vi "RedoCurveFits.vi"() -> ()   [LabVIEW 2020]
uses:
  <vilib>/Utility/file.llb/Read Delimited Spreadsheet (DBL).vi
  <vilib>/Utility/file.llb/Write Delimited Spreadsheet (DBL).vi
panel:
  out "XY Graph 5":cluster{dbl[], dbl[]}[](graph)
  out "error out":errorcluster
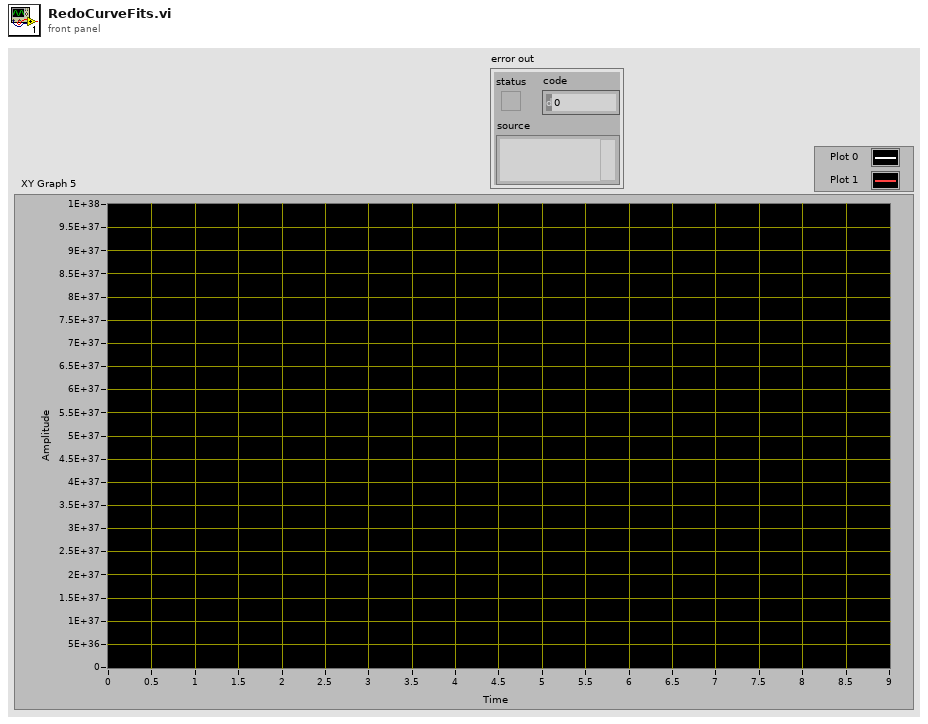
[diagram p1: front panel]
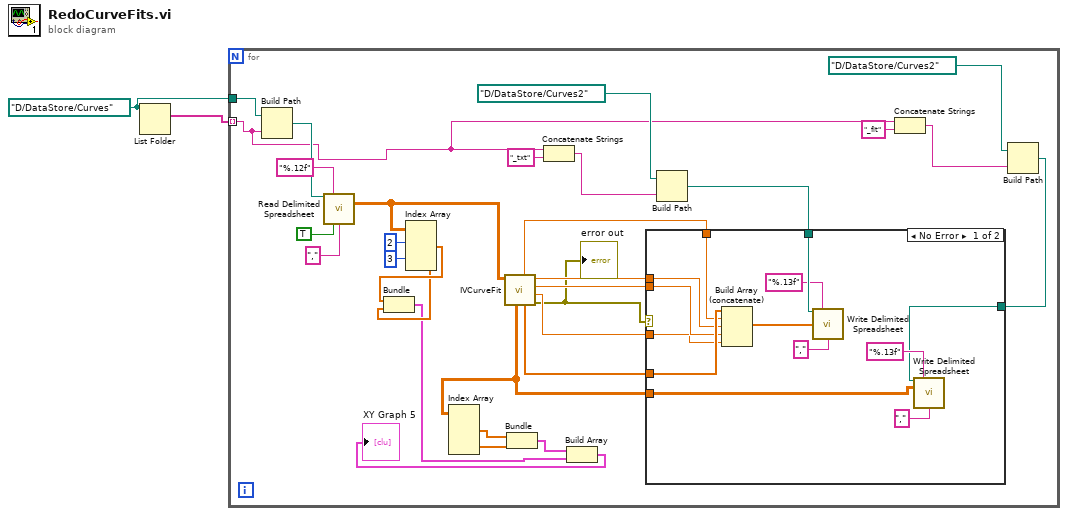
[diagram p0: block diagram]
diagram:
  w1 = path "D:/DataStore/Curves" ("path")
  n1 = List Folder(path=w1) -> (filenames=w2:string[])  [unwired: 3 in, 3 out]
  n2 = for {
    tunnel: w2 -> [w15] mode=indexing
    tunnel: w1 -> [w33]
    n3 = Build Path(base path=w33, name or relative path=w15) -> (appended path=w24:path)
    n4 = call-poly <vilib>:"Read Delimited Spreadsheet.vi"("file path (dialog if empty)"=w24, "format (%.3f)"="%.12f", "transpose? (F)"=TRUE, "delimiter (\\t)"="," ("delimiter (\\t)")) -> ("all rows"=w8:dbl[][])  [unwired: 6 in, 5 out]
    n5 = Index Array(array=w8, index (row) #1=2 ("index (row)"), index (row) #2=3 ("index (row)")) -> (element #1=w5:dbl[], element #2=w4:dbl[])  [unwired: 2 in]
    n6 = Bundle("all rows"=w5, "all rows"=w4) -> (w3:cluster{"all rows":dbl[], "all rows":dbl[]})  [unwired: 1 in]
    n7 = call "IVCurveFit.vi"("IVData"=w8) -> ("error out"=w20:errorcluster, "ChargeCapacitance"=w26:dbl, "Conductance"=w27:dbl, "Capacitance"=w28:dbl, "BestFit"=w29:dbl[], "residue"=w19:dbl, "Fit"=w13:dbl[][])  [unwired: 4 in]
    "error out" <- w20
    n8 = Index Array(array=w13) -> (element #1=w12:dbl[], element #2=w11:dbl[])  [unwired: 4 in]
    n9 = Bundle("Fit"=w12, "Fit"=w11) -> (w10:cluster{"Fit":dbl[], "Fit":dbl[]})  [unwired: 1 in]
    n10 = Concatenate Strings(w15, "_txt" ("string")) -> (w23:string)
    n11 = Build Array(w10, w3) -> (→"XY Graph 5":cluster{"all rows":dbl[], "all rows":dbl[]}[])
    n12 = Build Path(base path=path "D:/DataStore/Curves2", name or relative path=w23) -> (appended path=w22:path)
    n13 = Concatenate Strings(w15, "_fit" ("string")) -> (w17:string)
    n14 = Build Path(base path=path "D:/DataStore/Curves2", name or relative path=w17) -> (appended path=w14:path)
    n15 = case shown="No Error" w20 {
      tunnel: w29 -> [w46 _]
      tunnel: w28 -> [w45 _]
      tunnel: w27 -> [w44 _]
      tunnel: w26 -> [w43 _]
      tunnel: w22 -> [w41 _]
      tunnel: w19 -> [w38 _]
      tunnel: w14 -> [w35 _]
      tunnel: w13 -> [w34 _]
      frame No Error {
        n16 = Build Array (concatenate)(w46, w38, w45, w44, w43) -> (w42:dbl[])
        n17 = call-poly <vilib>:"Write Delimited Spreadsheet.vi"("file path (dialog if empty)"=w41, "format (%.3f)"="%.13f", "1D data"=w42, "delimiter (\\t)"="," ("delimiter (\\t)")) -> ()  [unwired: 10 in, 2 out]
        n18 = call-poly <vilib>:"Write Delimited Spreadsheet.vi"("file path (dialog if empty)"=w35, "format (%.3f)"="%.13f", "2D data"=w34, "delimiter (\\t)"="," ("delimiter (\\t)")) -> ()  [unwired: 10 in, 2 out]
      }
      frame Error {
      }
    }
  }
